vi "Execute Msg.vi"(7 "Actor in":refnum<class "Actor.lvclass">, 8 "Error in":errorcluster, 11 "Stopped Msg in":refnum<class "Stopped Msg.lvclass">) -> (0 "Error out":errorcluster, 2 "Msg Output":refnum<class "Msg Output.lvclass">, 5 "Actor out":refnum<class "Actor.lvclass">)   [LabVIEW 2025, in "jettl.lvlib" / "Stopped jettl Msg.lvlib" / "Stopped Msg.lvclass"]
uses:
  Stopped Msg.lvclass
  Actor/Actor.lvclass
  Msg Output/Msg Output.lvclass
  Stopped jettl Msg/Stopped jettl Msg.lvclass
  Stopped Msg.lvclass/Stopped Msg.ctl
  Stopped Msg Output/Stopped Msg Output.lvclass
  C:/git/jettl/src/jettl/jettl/Msg Output/Msg Output.lvclass
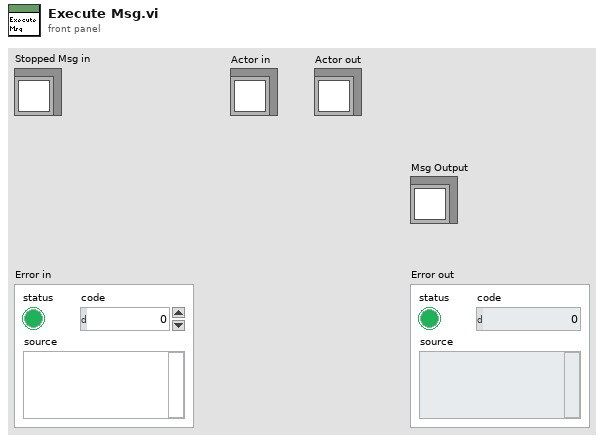
[diagram p1: front panel]
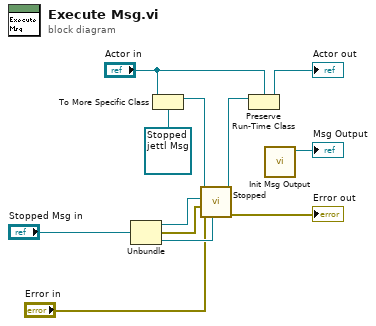
[diagram p0: block diagram]
diagram:
  n1 = Unbundle "Unbundle"("Stopped Msg in") -> (w5:refnum<class "Actor.lvclass">, w4:errorcluster, w3:refnum<class "Teller.lvclass">)
  n2 = To More Specific Class(target class=refnum<class "Stopped jettl Msg.lvclass"> refnum ("jettl.lvlib:jettl Msg Last Ack Creator Queue.lvlib:jettl Msg Last Ack Creator Queue.lvclass"), reference="Actor in") -> (specific class reference=w8:refnum<class "Stopped jettl Msg.lvclass">)  [unwired: 1 in, 1 out]
  n3 = call-dynamic "Stopped.vi"("Teller"=w3, "Error in"="Error in", "Error"=w4, "Actor"=w5, "Stopped jettl Msg in"=w8) -> ("Error out"=→"Error out":errorcluster, "Stopped jettl Msg out"=w7:refnum<class "Stopped jettl Msg.lvclass">)  [unwired: 5 in]
  n4 = Preserve Run-Time Class(object in=w7, 2:"Actor in") -> (object out=→"Actor out":refnum<class "Actor.lvclass">)  [unwired: 1 in, 1 out]
  n5 = call "Init Msg Output.vi"() -> ("Stopped Msg Output out"=→"Msg Output":refnum<class "Stopped Msg Output.lvclass">)  [unwired: 11 in]
